vi "Get User Roles.vi"(8 "error in (no error)":errorcluster, 10 "Username":string, 11 "I Authentication Provider in":refnum<class "I Authentication Provider.lvclass">) -> (0 "error out":errorcluster, 2 "User roles":T1[](array[typedef]), 3 "I Authentication Provider out":refnum<class "I Authentication Provider.lvclass">)   [LabVIEW 2026, in "I Authentication Provider.lvclass"]
uses:
  I Authentication Provider.lvclass
  Typedefs/enums/Role Enum.ctl
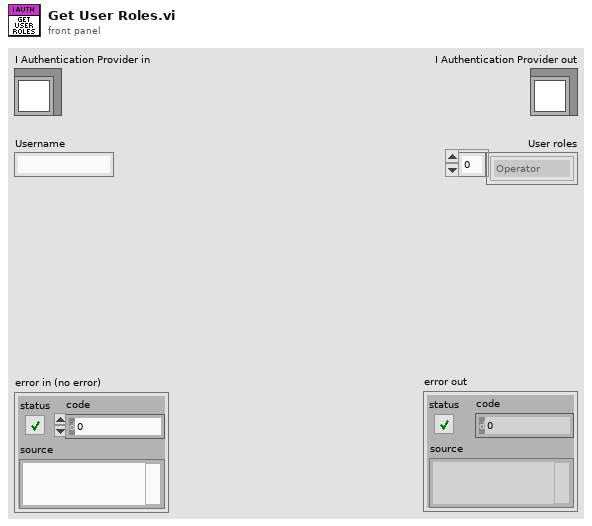
[diagram p1: front panel]
types:
  T1 = typedef "Role Enum.ctl" = enum16{"Operator", "Engineer", "Admin"}
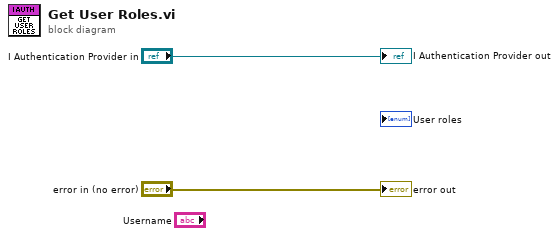
[diagram p0: block diagram]
diagram:
  "I Authentication Provider out" <- "I Authentication Provider in"
  "error out" <- "error in (no error)"
